vi "oa_AC DC Separation Linear (N Channel).vi"(7 "reset? (F)":bool, 8 "points/rev":u32, 9 "averaging revolution (1)":dbl=1.0 min=0.0, 10 "position info":T1, 11 "even angle signals":cluster{"r0":dbl, "dr":dbl, "Y":dbl[]}[](array[cluster]) {"r0" format="%.2p"; "dr" format="%.2p"; "Y" format="%.2f"}) -> (0 "DC even angle signals":cluster{"r0":dbl, "dr":dbl, "Y":dbl[]}[](array[cluster]), 1 "AC even angle signals":cluster{"r0":dbl, "dr":dbl, "Y":dbl[]}[](array[cluster]), 2 "position info out":T1, 3 "dul even angle signals":cluster{"r0":dbl, "dr":dbl, "Y":dbl[]}[](array[cluster]))   [LabVIEW 2017, in "SoundVib_OAUtility.lvlib"]
uses:
  <vilib>/addons/Sound and Vibration/Order Analysis/Utility/SoundVib_OAUtility.lvlib
  <vilib>/addons/Sound and Vibration/Order Analysis/Misc/OAT Position Info.ctl
  <vilib>/Analysis/baseanly.llb/Mean (DBL).vi
  <vilib>/Analysis/NI_AALBase.lvlib
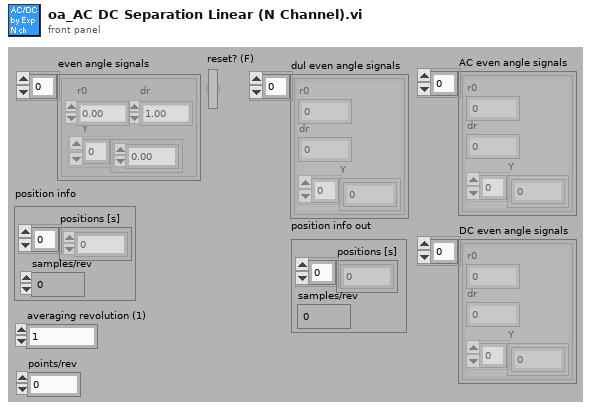
[diagram p1: front panel]
types:
  T1 = typedef "OAT Position Info.ctl" = cluster{"positions [s]":dbl[], "samples/rev":dbl}
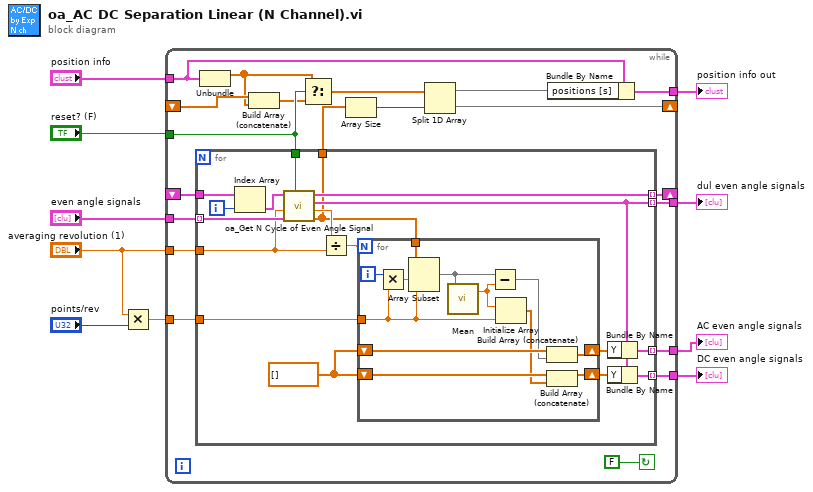
[diagram p0: block diagram]
diagram:
  n1 = Multiply(x="averaging revolution (1)", y="points/rev") -> (x*y=w3:dbl)
  n2 = while {
    tunnel: "even angle signals" -> [w29]
    tunnel: "reset? (F)" -> [w21]
    shift-right: [w27] -> _
    shift-left: _ -> [w28]
    tunnel: w3 -> [w26]
    tunnel: [w25] -> w7
    tunnel: [w24] -> w6
    tunnel: [w23] -> w8
    tunnel: "averaging revolution (1)" -> [w22]
    tunnel: "position info" -> [w14]
    shift-right: [w12] -> _
    shift-left: _ -> [w19]
    tunnel: [w11] -> w1
    stop <- FALSE continue-if-true
    n3 = for {
      tunnel: w29 -> [w40] mode=indexing
      tunnel: w21 -> [w39]
      tunnel: w28 -> [w47]
      tunnel: [w38] -> w27 mode=indexing
      tunnel: w26 -> [w45]
      tunnel: [w44] -> w25 mode=indexing
      tunnel: [w42] -> w24 mode=indexing
      tunnel: [w36] -> w23 mode=indexing
      tunnel: w22 -> [w32]
      tunnel: [w31] -> w20
      i -> [w46]
      w41 = dbl[] [] ("second subarray")
      n4 = Index Array(array=w47, index=w46) -> (element=w37:cluster{"r0":dbl, "dr":dbl, "Y":dbl[]})
      n5 = call <vilib>:"oa_Get N Cycle of Even Angle Signal.vi"("reset"=w39, "new even angle signal"=w40, "averaging revolution (1)"=w32, "rest even angle signal"=w37) -> ("data for averaging"=w31:dbl[], "number of averages"=w34:dbl, "even angle signal"=w36:cluster{"r0":dbl, "dr":dbl, "Y":dbl[]}, "rest even angle signal out"=w38:cluster{"r0":dbl, "dr":dbl, "Y":dbl[]})  [unwired: 4 in]
      n6 = Divide(x=w34, y=w32) -> (x/y=w33:dbl)
      n7 = for {
        N: w33 -> [_]
        tunnel: w45 -> [w49]
        shift-right: [w57] -> w35
        shift-left: w41 -> [w59]
        shift-right: [w53] -> w43
        shift-left: w41 -> [w55]
        tunnel: w31 -> [w52]
        i -> [w50]
        n8 = Multiply(x=w50, y=w49) -> (x*y=w48:dbl)
        n9 = Array Subset(array=w52, index=w48, length=w49) -> (w51:dbl[])
        n10 = call-poly <vilib>:"Mean.vi"("X"=w51) -> ("mean"=w56:dbl)  [unwired: 1 out]
        n11 = Subtract(x=w51, y=w56) -> (x-y=w58:dbl[])
        n12 = Initialize Array(w56, w49) -> (w54:dbl[])
        n13 = Build Array (concatenate)(w59, w58) -> (w57:dbl[])
        n14 = Build Array (concatenate)(w55, w54) -> (w53:dbl[])
      }
      n15 = Bundle By Name(cluster=w36, "Y"=w35) -> (w44:cluster{"r0":dbl, "dr":dbl, "Y":dbl[]})
      n16 = Bundle By Name(cluster=w36, "Y"=w43) -> (w42:cluster{"r0":dbl, "dr":dbl, "Y":dbl[]})
    }
    n17 = Unbundle(w14) -> ("positions [s]"=w18:dbl[])  [unwired: 1 out]
    n18 = Build Array (concatenate)(w19, w18) -> (w17:dbl[])
    n19 = Select(t=w18, s=w21, f=w17) -> (s? t:f=w16:dbl[])
    n20 = Array Size(array=w20) -> (size(s)=w15:i32)
    n21 = Split 1D Array(array=w16, index=w15) -> (first subarray=w13:dbl[], second subarray=w12:dbl[])
    n22 = Bundle By Name(cluster=w14, "positions [s]"=w13) -> (w11:T1)
  }
  "dul even angle signals" <- w8
  "AC even angle signals" <- w7
  "DC even angle signals" <- w6
  "position info out" <- w1
